vi "Umgebung.Strahlungsleistung.vi"(8 "Error in":errorcluster, 11 "Umgebung in":refnum<data-value>) -> (0 "Error out":errorcluster, 3 "Umgebung out":refnum<data-value>)   [LabVIEW 2016, in "Umgebung.lvclass"]
uses:
  Umgebung.lvclass
  Umgebung.lvclass/Umgebung.ctl
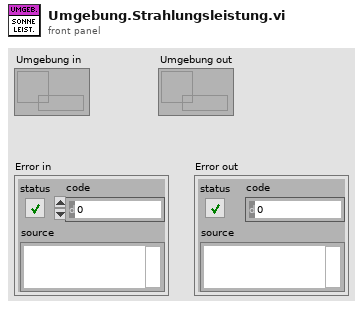
[diagram p1: front panel]
types:
  T1 = enum16{"Klarer Himmel", "Leichte Bewölkung", "Starke Bewölkung"}
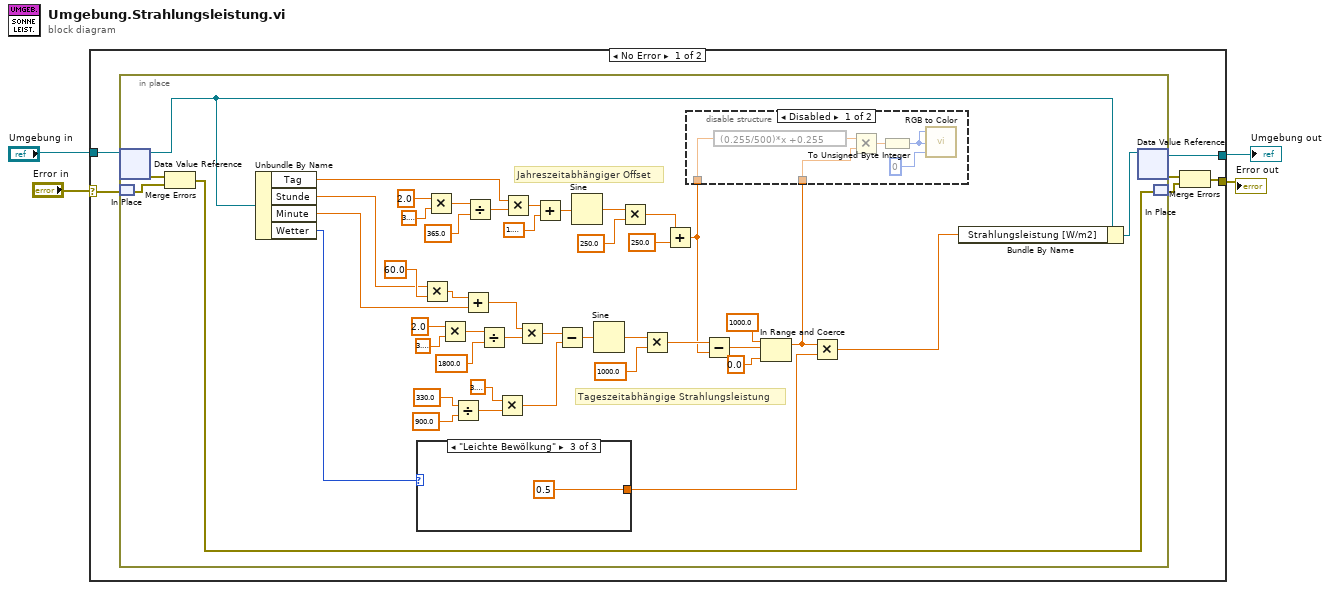
[diagram p0: block diagram]
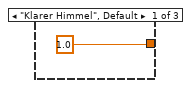
[diagram p2: hidden frame]
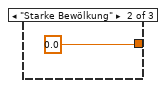
[diagram p3: hidden frame]
diagram:
  n1 = case shown="No Error" "Error in" {
    selector: "Error in" -> [w7 w67]
    tunnel: [w8 w67] -> w2
    tunnel: [w10 w66] -> w3
    tunnel: "Umgebung in" -> [w5 w66]
    frame No Error {
      n2 = in-place {
        # "Tageszeitabhängige Strahlungsleistung"
        # "Jahreszeitabhängiger Offset"
        n3 = in-place-dvr #1(w5) -> (w53:refnum<class "Umgebung.lvclass">, w55:errorcluster)
        n4 = in-place-match #2(w7) -> (w54:errorcluster)
        n5 = Merge Errors(w55, w54) -> (w56:errorcluster)
        n6 = Unbundle By Name(w53) -> ("Tag"=w44:dbl, "Stunde"=w17:dbl, "Minute"=w37:dbl, "Wetter"=w13:T1)
        n7 = case shown="\"Leichte Bewölkung\"" w13 {
          tunnel: [1.0 0.0 0.5] -> w12
          frame "Klarer Himmel", Default {
          }
          frame "Starke Bewölkung" {
          }
          frame "Leichte Bewölkung" {
          }
        }
        n8 = Multiply(x=w17, y=60.0) -> (x*y=w38:dbl)
        n9 = Multiply(x=2.0, y=3.141592653589793) -> (x*y=w48:dbl)
        n10 = Multiply(x=2.0, y=3.141592653589793) -> (x*y=w33:dbl)
        n11 = Divide(x=330.0 ("y"), y=900.0) -> (x/y=w28:dbl)
        n12 = Add(x=w38, y=w37) -> (x+y=w29:dbl)
        n13 = Divide(x=w48, y=365.0) -> (x/y=w46:dbl)
        n14 = Divide(x=w33, y=1800.0) -> (x/y=w31:dbl)
        n15 = Multiply(x=3.141592653589793, y=w28) -> (x*y=w23:dbl)
        n16 = Multiply(x=w44, y=w46) -> (x*y=w42:dbl)
        n17 = Multiply(x=w29, y=w31) -> (x*y=w24:dbl)
        n18 = Add(x=w42, y=1.5707963267948966) -> (x+y=w40:dbl)
        n19 = Subtract(x=w24, y=w23) -> (x-y=w22:dbl)
        n20 = Sine(x=w40) -> (sin(x)=w50:dbl)
        n21 = Sine(x=w22) -> (sin(x)=w35:dbl)
        n22 = Multiply(x=w50, y=250.0) -> (x*y=w52:dbl)
        n23 = Multiply(x=w35, y=1000.0) -> (x*y=w21:dbl)
        n24 = Add(x=w52, y=250.0) -> (x+y=w16:dbl)
        n25 = Subtract(x=w21, y=w16) -> (x-y=w18:dbl)
        n26 = In Range and Coerce(upper limit=1000.0, x=w18, lower limit=0.0) -> (coerced(x)=w14:dbl)  [unwired: 1 out]
        n27 = disable-structure shown="Disabled" {
          disable-tunnel: w16 -> [w65 _]
          disable-tunnel: w14 -> [w60 _]
          frame Disabled {
            n28 = expression code="(0.255/500)*x +0.255"(w65) -> (w61:dbl)
            n29 = Multiply(x=w61, y=w60) -> (x*y=w64:dbl)
            n30 = To Unsigned Byte Integer(number=w64) -> (unsigned 8bit integer=w63:u8)
            n31 = call <vilib>:"RGB to Color.vi"("B"=u8 0, "G"=w63, "R"=w63) -> ()  [unwired: 1 out]
          }
          frame Enabled {
          }
        }
        n32 = Multiply(x=w14, y=w12) -> (x*y=w11:dbl)
        n33 = Bundle By Name(cluster=w53, "Strahlungsleistung [W/m2]"=w11) -> (w15:refnum<class "Umgebung.lvclass">)
        n34 = in-place-dvr #1(w15) -> (w10:refnum<data-value>, w9:errorcluster)
        n35 = in-place-match #2(w56) -> (w6:errorcluster)
      }
      n36 = Merge Errors(w9, w6) -> (w8:errorcluster)
    }
    frame Error {
    }
  }
  "Umgebung out" <- w3
  "Error out" <- w2
